vi "StopProcess.vi"(0 "reference in":refnum<class "Dynamic.lvclass">, 2 "ms timeout (-1)":i32=-1, 5 "error in (no error)":errorcluster) -> (14 "reference out":refnum<class "Dynamic.lvclass">, 19 "error out":errorcluster)   [LabVIEW 2019, in "Dynamic.lvclass"]
uses:
  Dynamic.lvclass
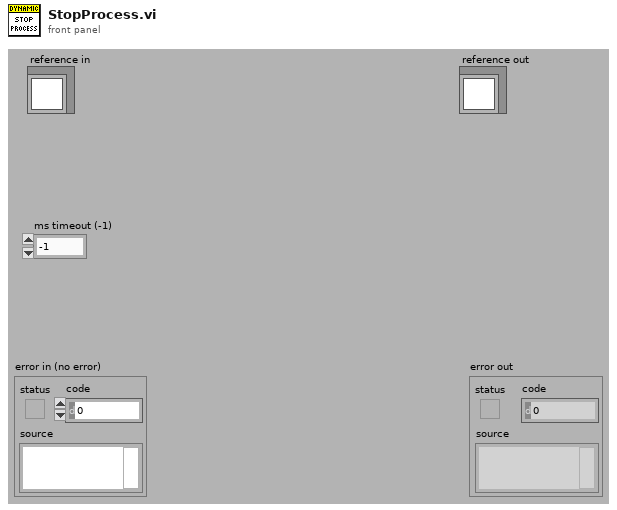
[diagram p1: front panel]
types:
  T1 = enum16{"ReadRepository", "CreateNew", "CreateOrLookUpExisting", "ReadRepositoryAndDestroy"}
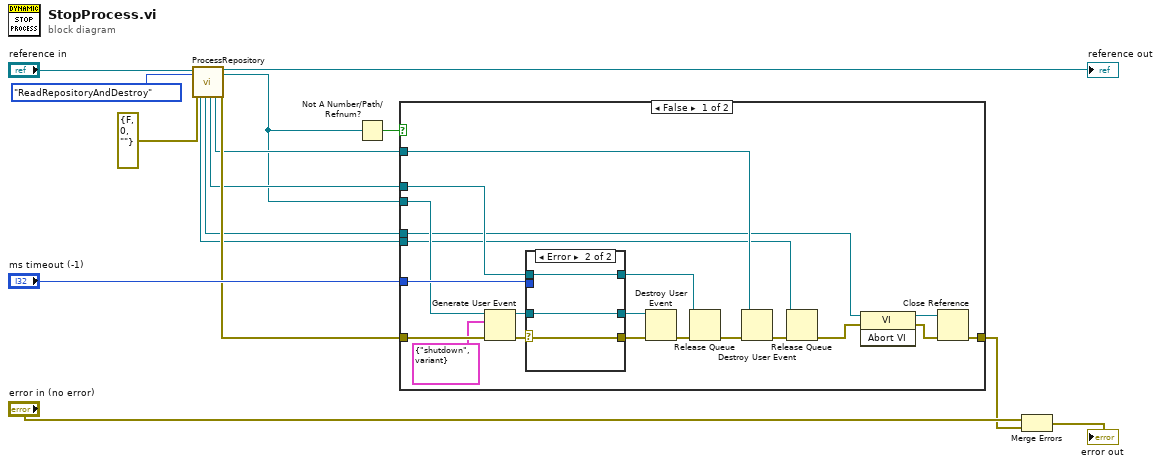
[diagram p0: block diagram]
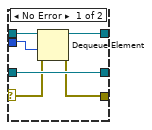
[diagram p2: hidden frame]
diagram:
  n1 = call "ProcessRepository.vi"("reference in"="reference in", "Action(ReadRepository)"=T1."ReadRepositoryAndDestroy", "error in (no error)"=errorcluster {"status"=FALSE, "code"=0, "source"=""}) -> ("QueueFromProcess"=w2:refnum<queue>, "ProcessViRef"=w6:refnum<vi>, "ProcessSyncQueue"=w8:refnum<queue>, "EventFromProcess"=w7:refnum<user-event>, "reference out"=→"reference out":refnum<class "Dynamic.lvclass">, "EventsToProcess"=w4:refnum<user-event>, "error out"=w9:errorcluster)  [unwired: 9 in, 1 out]
  n2 = Not A Number/Path/Refnum?(number/path/refnum=w4) -> (NaN/Path/Refnum?=w3:bool)
  n3 = case shown="False" w3 {
    tunnel: w8 -> [w35 _]
    tunnel: w9 -> [w27 w45]
    tunnel: [w31 w45] -> w13
    tunnel: w4 -> [w26 _]
    tunnel: "ms timeout (-1)" -> [w30 _]
    tunnel: w7 -> [w28 _]
    tunnel: w6 -> [w24 _]
    tunnel: w2 -> [w20 _]
    frame False {
      n4 = Generate User Event(user event=w26, event data cluster=cluster{"Command":string, "Data":variant} {"Command"="shutdown", "Data"=variant} ("event data"), error in=w27) -> (user event out=w34:refnum<user-event>, error out=w29:errorcluster)  [unwired: 1 in]
      n5 = case shown="Error" w29 {
        tunnel: [w39 w44] -> w33
        tunnel: w35 -> [w38 w42]
        tunnel: [w41 w43] -> w32
        tunnel: w34 -> [w41 w43]
        tunnel: w30 -> [w37 _]
        selector: w29 -> [w40 w44]
        tunnel: [w36 w42] -> w16
        frame No Error {
          n6 = Dequeue Element(queue=w38, timeout in ms (-1)=w37, error in (no error)=w40) -> (queue out=w36:refnum<queue>, error out=w39:errorcluster)  [unwired: 2 out]
        }
        frame Error {
        }
      }
      n7 = Destroy User Event(user event=w32, error in=w33) -> (error out=w18:errorcluster)
      n8 = Release Queue(queue=w16, error in (no error)=w18) -> (error out=w17:errorcluster)  [unwired: 1 in, 2 out]
      n9 = Destroy User Event(user event=w28, error in=w17) -> (error out=w21:errorcluster)
      n10 = Release Queue(queue=w20, error in (no error)=w21) -> (error out=w19:errorcluster)  [unwired: 1 in, 2 out]
      n11 = invoke class="VI" method="Abort VI"(reference=w24, error in=w19) -> (reference out=w23:refnum<vi>, error out=w22:errorcluster)  [unwired: 1 in, 1 out]
      n12 = Close Reference(reference=w23, error in (no error)=w22) -> (error out=w31:errorcluster)
    }
    frame True {
    }
  }
  n13 = Merge Errors("error in (no error)", w13) -> (→"error out":errorcluster)
